vi "Send Message over UDP.vi"(0 "message":T1, 1 "UDP receiver port (if not found)":u16, 5 "UDP connection ID":refnum<k16>, 9 "timeout (25000 ms)":i32=25200, 11 "error in":errorcluster) -> (6 "message string":string, 10 "timed out?":bool, 15 "error out":errorcluster)   [LabVIEW 2014, in "AMC.lvlib"]
doc: "Sends a message to a receiver process over UDP.\n\nIf <b>UDP connection ID</b> is wired, the message will be sent using that connection.\n\nIf <b>UDP connection ID</b> is unwired, the message will be sent using the same connection as <b>UDP Dispatcher.vi</b>."
uses:
  AMC.lvlib
  Message.ctl
  <vilib>/NI/Tools/Keyed Array/KeyedArray.ctl
  <vilib>/NI/Tools/Keyed Array/Tools_KeyedArray.lvlib
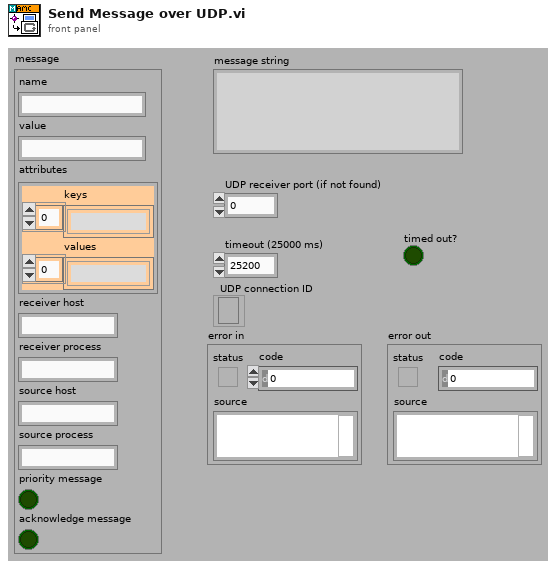
[diagram p1: front panel]
types:
  T1 = typedef "AMC.lvlib/Message.ctl" = cluster{"name":string, "value":string, "attributes":T2, "receiver host":string, "receiver process":string, "source host":string, "source process":string, "priority message":bool, "acknowledge message":bool}
  T2 = typedef "Tools_KeyedArray.lvlib/KeyedArray.ctl" = cluster{"keys":string[], "values":string[]}
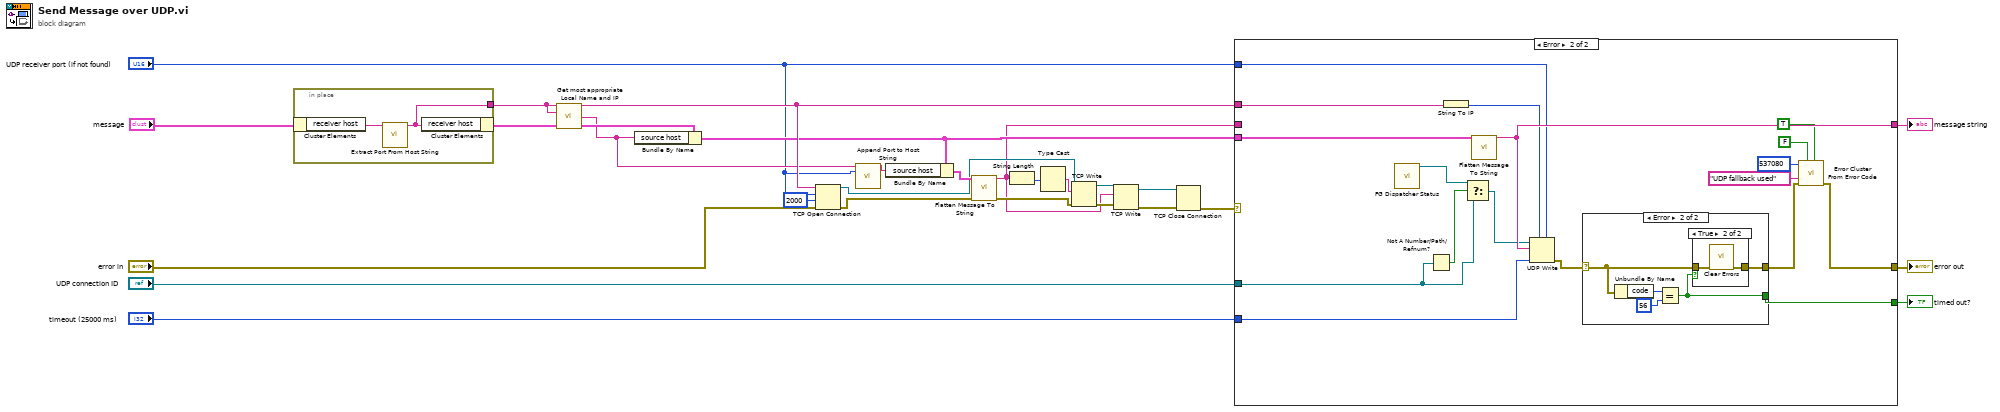
[diagram p0: block diagram]
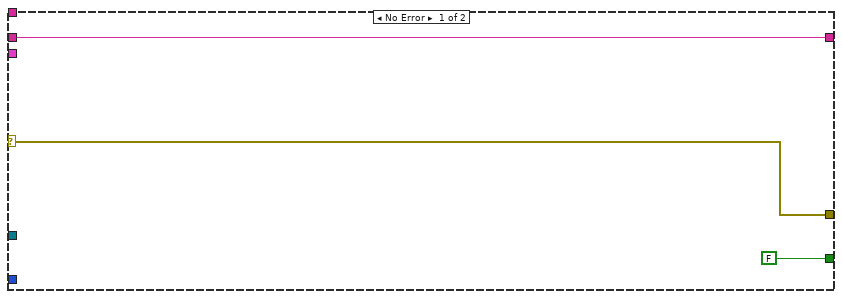
[diagram p2: hidden frame]
diagram:
  n1 = in-place {
    in-place-border: [w27] -> w19
    n2 = in-place-cluster #1("message") -> ("receiver host"=w28:string)
    n3 = call "Extract Port From Host String.vi"("host in"=w28) -> ("host out"=w27:string)  [unwired: 12 in, 2 out]
    n4 = in-place-cluster #1("receiver host"=w27) -> (w20:T1)
  }
  n5 = call "Get most appropriate Local Name and IP.vi"("target host"=w19) -> ("best source IP"=w15:string)  [unwired: 14 in]
  n6 = Bundle By Name(cluster=w20, "source host"=w15) -> (w17:T1)
  n7 = TCP Open Connection(address=w19, remote port or service name="UDP receiver port (if not found)", timeout ms (60000)=2000, error in (no error)="error in") -> (connection ID=w9:refnum<k5>, error out=w12:errorcluster)  [unwired: 1 in]
  n8 = call "Append Port to Host String.vi"("host in"=w15, "port"="UDP receiver port (if not found)") -> ("host out"=w16:string)  [unwired: 13 in]
  n9 = Bundle By Name(cluster=w17, "source host"=w16) -> (w13:T1)
  n10 = call "Flatten Message To String.vi"("message"=w13, "error in"=w12) -> ("message string"=w1:string, "error out"=w8:errorcluster)  [unwired: 12 in]
  n11 = String Length(string=w1) -> (length=w11:i32)
  n12 = Type Cast(x=w11) -> (*(type *) &x=w10:string)  [unwired: 1 in]
  n13 = TCP Write(connection ID=w9, data in=w10, error in (no error)=w8) -> (connection ID out=w6:refnum<k5>, error out=w7:errorcluster)  [unwired: 1 in, 1 out]
  n14 = TCP Write(connection ID=w6, data in=w1, error in (no error)=w7) -> (connection ID out=w4:refnum<k5>, error out=w3:errorcluster)  [unwired: 1 in, 1 out]
  n15 = TCP Close Connection(connection ID=w4, error in (no error)=w3) -> (error out=w2:errorcluster)  [unwired: 1 in, 1 out]
  n16 = case shown="Error" w2 {
    selector: w2 -> [w30 _]
    tunnel: [w30 w32] -> w26
    tunnel: "timeout (25000 ms)" -> [_ w49]
    tunnel: [w31 w48] -> w23
    tunnel: [FALSE w47] -> w22
    tunnel: "UDP connection ID" -> [_ w46]
    tunnel: w19 -> [_ w41]
    tunnel: w17 -> [_ w40]
    tunnel: "UDP receiver port (if not found)" -> [_ w39]
    tunnel: w1 -> [w31 _]
    frame No Error {
    }
    frame Error {
      n17 = call "FG Dispatcher Status.vi"() -> ("UDP connection ID"=w43:refnum<k16>)  [unwired: 13 in, 2 out]
      n18 = Not A Number/Path/Refnum?(number/path/refnum=w46) -> (NaN/Path/Refnum?=w44:bool)
      n19 = String To IP(1:w41) -> (0:w45:u32)
      n20 = Select(t=w43, s=w44, f=w46) -> (s? t:f=w42:refnum<k16>)
      n21 = call "Flatten Message To String.vi"("message"=w40) -> ("message string"=w48:string)  [unwired: 13 in, 1 out]
      n22 = UDP Write(address=w45, port or service name=w39, connection ID=w42, data in=w48, 9:w49) -> (error out=w34:errorcluster)  [unwired: 1 in, 1 out]
      n23 = case shown="Error" w34 {
        selector: w34 -> [w50 w53]
        tunnel: [w50 w52] -> w33
        tunnel: [_ w51] -> w47
        frame No Error {
        }
        frame Error {
          n24 = Unbundle By Name(w53) -> ("code"=w55:i32)
          n25 = Equal?(x=w55, y=56) -> (x = y?=w51:bool)
          n26 = case shown="True" w51 {
            tunnel: w53 -> [w56 w58]
            tunnel: [w56 w57] -> w52
            frame False {
            }
            frame True {
              n27 = call <vilib>:"Clear Errors.vi"("error in (no error)"=w58) -> ("error out"=w57:errorcluster)  [unwired: 5 in, 1 out]
            }
          }
        }
      }
      n28 = call <vilib>:"Error Cluster From Error Code.vi"("is warning? (False)"=TRUE, "show call chain? (False)"=FALSE, "error in (no error)"=w33, "error message (\"\")"="UDP fallback used" ("error message (\"\")"), "error code (0)"=537080) -> ("error out"=w32:errorcluster)  [unwired: 4 in]
    }
  }
  "error out" <- w26
  "message string" <- w23
  "timed out?" <- w22
